vi "Release Semaphore.vi"(4 "error in (no error)":errorcluster, 7 "semaphore":T1) -> (0 "error out":errorcluster, 3 "semaphore out":T1)   [LabVIEW 2013]
doc: "Releases access to a semaphore. If the Acquire Semaphore VI is waiting for the semaphore this VI releases, it stops waiting and continues execution."
uses:
  Semaphore Refnum Core.ctl
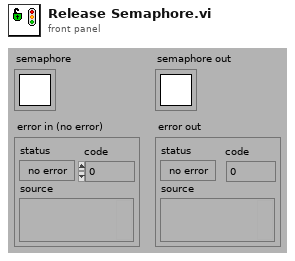
[diagram p1: front panel]
types:
  T1 = typedef "Semaphore RefNum" = refnum<k1>
  T2 = typedef "Semaphore Refnum Core.ctl" = refnum<k1>
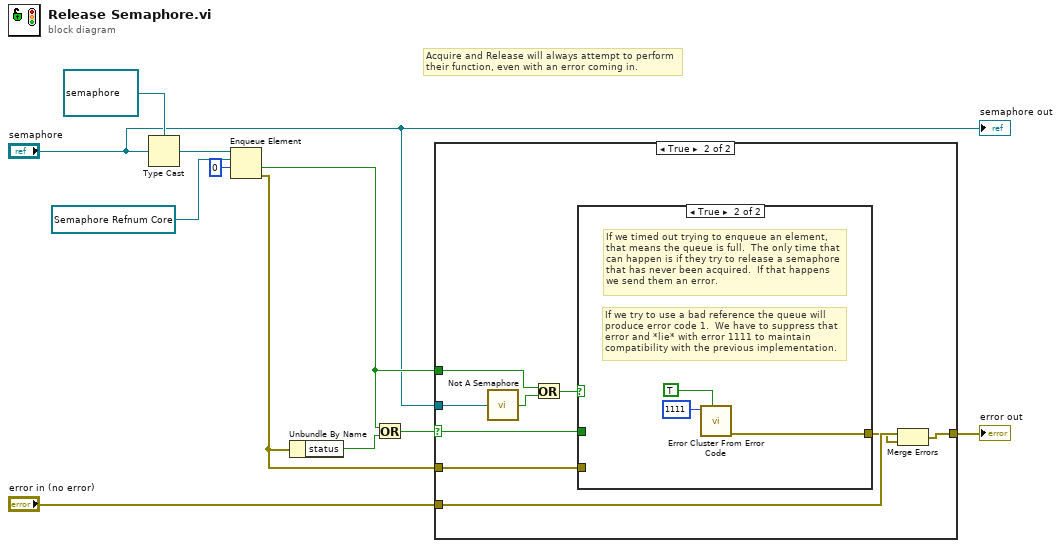
[diagram p0: block diagram]
diagram:
  w8 = T2 refnum items=["Semaphore Core"] ("element")
  w11 = refnum<queue> refnum items=["Semaphore Core"] ("queue out")
  # "Acquire and Release will always attempt to perform their function, even with an error coming in."
  n1 = Type Cast(type=w11, x="semaphore") -> (*(type *) &x=w10:refnum<queue>)
  n2 = Enqueue Element(queue=w10, element=w8, timeout in ms (-1)=0) -> (timed out?=w3:bool, error out=w1:errorcluster)  [unwired: 1 in, 1 out]
  n3 = Unbundle By Name(w1) -> ("status"=w6:bool)
  n4 = Or(x=w3, y=w6) -> (x .or. y?=w7:bool)
  n5 = case shown="True" w7 {
    selector: w7 -> [_ w21]
    tunnel: [w12 w13] -> w4
    tunnel: "error in (no error)" -> [w12 w15]
    tunnel: w3 -> [_ w20]
    tunnel: "semaphore" -> [_ w19]
    tunnel: w1 -> [_ w18]
    frame False {
    }
    frame True {
      n6 = call "Not A Semaphore.vi"("semaphore"=w19) -> ("not a semaphore"=w17:bool)
      n7 = Or(x=w20, y=w17) -> (x .or. y?=w16:bool)
      n8 = case shown="True" w16 {
        tunnel: w21 -> [_ _]
        tunnel: [w22 w23] -> w14
        tunnel: w18 -> [w22 _]
        frame False {
        }
        frame True {
          # "If we timed out trying to enqueue an element, that means the queue is full.  The only time that can happen is if they try to release a semaphore that has never been acquired.  If that happens we send them an error."
          # "If we try to use a bad reference the queue will produce error code 1.  We have to suppress that error and *lie* with error 1111 to maintain compatibility with the previous implementation."
          n9 = call "Error Cluster From Error Code.vi"("show call chain? (False)"=TRUE, "error code (0)"=1111 ("code")) -> ("error out"=w23:errorcluster)  [unwired: 1 in, 6 out]
        }
      }
      n10 = Merge Errors(w15, w14) -> (w13:errorcluster)
    }
  }
  "error out" <- w4
  "semaphore out" <- "semaphore"
